vi "Get Library and Member Name.vi"(10 "Fully Qualified Name":string) -> (1 "Name":string, 2 "Package":string)   [LabVIEW 2013, in "JUnit Conversion.lvlib"]
uses:
  JUnit Conversion.lvlib
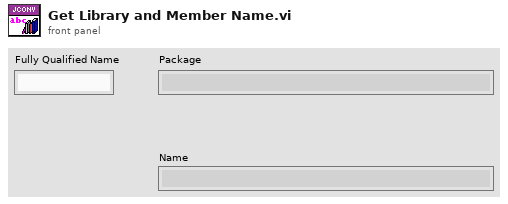
[diagram p1: front panel]
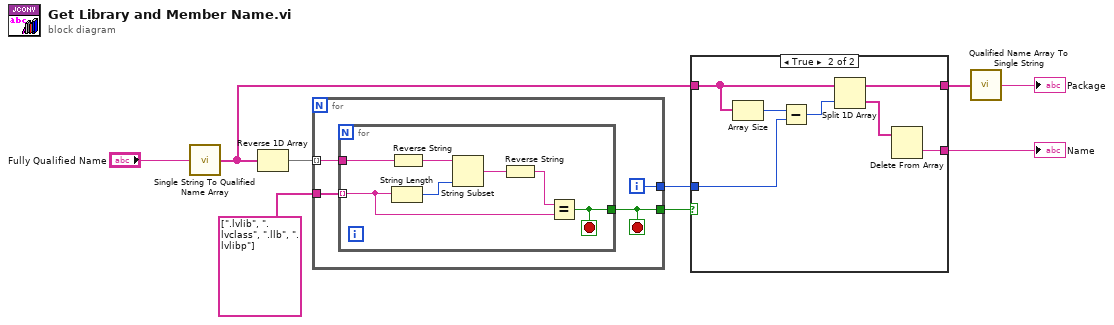
[diagram p0: block diagram]
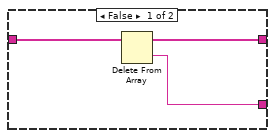
[diagram p2: hidden frame]
diagram:
  n1 = call <vilib>:"Single String To Qualified Name Array.vi"("Fully Qualified String"="Fully Qualified Name") -> ("Fully Qualified Array"=w2:string[])
  n2 = Reverse 1D Array(array=w2) -> (reversed array=w8:string[])
  n3 = for {
    tunnel: w8 -> [w12] mode=indexing
    tunnel: string[] [".lvlib", ".lvclass", ".llb", ".lvlibp"] -> [w13]
    tunnel: [w11] -> w6
    tunnel: [w10] -> w7
    i -> [w10]
    stop <- w11 stop-if-true
    n4 = for {
      tunnel: w13 -> [w15] mode=indexing
      tunnel: w12 -> [w20]
      tunnel: [w14] -> w11
      stop <- w14 stop-if-true
      n5 = String Length(string=w15) -> (length=w18:i32)
      n6 = Reverse String(1:w20) -> (0:w19:string)
      n7 = String Subset(string=w19, length (rest)=w18) -> (substring=w17:string)  [unwired: 1 in]
      n8 = Reverse String(1:w17) -> (0:w16:string)
      n9 = Equal?(x=w16, y=w15) -> (x = y?=w14:bool)
    }
  }
  n10 = case shown="True" w6 {
    tunnel: w2 -> [w23 w30]
    tunnel: w7 -> [_ w24]
    tunnel: [w22 w27] -> w5
    tunnel: [w21 w25] -> w1
    frame False {
      n11 = Delete From Array(array=w23) -> (deleted portion=w21:string, array with subset deleted=w22:string[])  [unwired: 2 in]
    }
    frame True {
      n12 = Array Size(array=w30) -> (size(s)=w29:i32)
      n13 = Subtract(x=w29, y=w24) -> (x-y=w28:i32)
      n14 = Split 1D Array(array=w30, index=w28) -> (first subarray=w27:string[], second subarray=w26:string[])
      n15 = Delete From Array(array=w26) -> (deleted portion=w25:string)  [unwired: 2 in, 1 out]
    }
  }
  "Name" <- w1
  n16 = call <vilib>:"Qualified Name Array To Single String.vi"("Fully Qualified Array"=w5) -> ("Fully Qualified String"=→"Package":string)
